vi "USB6363_Output_demo.vi"() -> ()   [LabVIEW 2013]
doc: "This example demonstrates how to continuously re-generate analog output data from a buffer in your computer's memory.\n\nRefer to your device documentation for pinouts and hardware capabilities."
uses:
  <vilib>/Utility/error.llb/DialogType.ctl
  <vilib>/DAQmx/create/channels.llb/DAQmx Create Channel (AO-Voltage-Basic).vi
  <vilib>/DAQmx/configure/timing.llb/DAQmx Timing (Sample Clock).vi
  <vilib>/DAQmx/write.llb/DAQmx Write (Analog 1D Wfm NChan NSamp).vi
  <vilib>/DAQmx/configure/trigger.llb/DAQmx Start Trigger (Digital Edge).vi
  <vilib>/DAQmx/configure/trigger.llb/DAQmx Start Trigger (Analog Edge).vi
  <resource>/objmgr/daqmx.rc
panel:
  in  "Waveform settings":T1={"Tx"=0.3, "Vx_max"=1.0, "Vy_max"=1.0, "Row_N"=20, "ratio of decline"=0.3}
  in  "Trigger Type":T2(tab)
  in  "Edge":i32(ring)=10280 items=["Rising"=10280, "Falling"=10171]
  in  "Digital Trigger Source":tag
  in  "Level (V)":dbl format="%0.2f"
  in  "Hysteresis (V)":dbl
  in  "Slope":i32(ring)=10280 items=["Rising"=10280, "Falling"=10171]
  in  "Analog Trigger Source":string="APFI0"
  in  "Pause When":i32(ring)=10192 items=["High"=10192, "Low"=10214]
  in  "Pause Trigger Source":tag
  in  "Stop":bool
  out "Waveform Graph":waveform(dbl)[](graph)
  in  "Sample Rate":dbl=1000.0
  in  "Sample Clock Source":tag="OnboardClock"
  in  "Max Voltage":dbl=5.0
  in  "Min Voltage":dbl=-5.0
  in  "Physical Channel(s)":tag="Dev1/ao2:3"
  out "Actual Sample Rate":dbl=1000.0 format="%0.2f"
  # "Channel Settings"
  # "Output"
  # "Timing and Buffer Settings"
  # "Trigger Settings"
  # "Waveform Settings"
  # "The number of elements in the waveform array must equal the number of channels in the task."
  # "To configure and use a start trigger you must have the necessary tab selected above.  Not all hardware supports triggering--refer to your device documentation for more info."
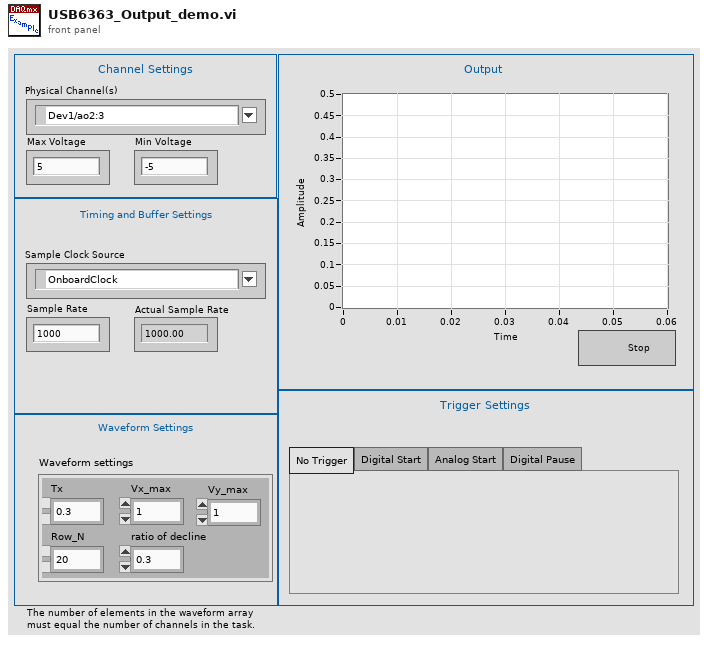
[diagram p1: front panel]
types:
  T1 = cluster{"Tx":dbl, "Vx_max":dbl, "Vy_max":dbl, "Row_N":i32, "ratio of decline":dbl}
  T2 = enum32{"No Trigger", "Digital Start", "Analog Start", "Digital Pause"}
  T3 = typedef "DialogType.ctl" = u16
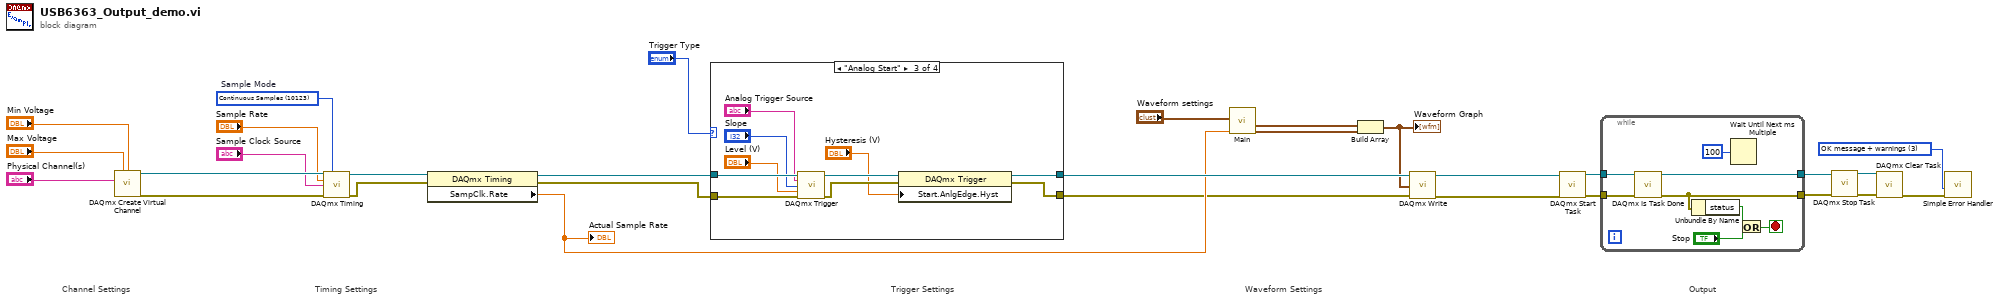
[diagram p0: block diagram]
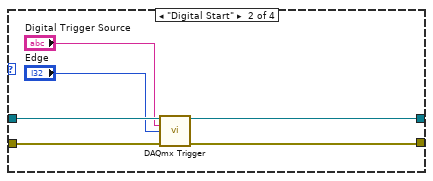
[diagram p3: hidden frame]
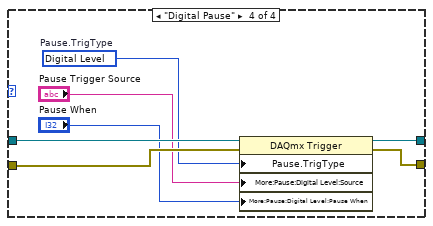
[diagram p4: hidden frame]
diagram:
  w7 = T3 3 items=["no dialog", "OK message", "continue or stop message", "OK message + warnings", "continue/stop + warnings"] ("type of dialog (OK msg:1)")
  w28 = 10123 items=["Finite Samples"=10178, "Continuous Samples"=10123, "Hardware Timed Single Point"=12522]  # Sample Mode
  # "Output"
  # "Trigger Settings"
  # "Waveform Settings"
  # "Timing Settings"
  # "Channel Settings"
  n1 = call-poly <vilib>:"DAQmx Create Virtual Channel.vi"("maximum value"="Max Voltage", "minimum value"="Min Voltage", "physical channels"="Physical Channel(s)") -> ("task out"=w26:refnum<k21>, "error out"=w27:errorcluster)  [unwired: 11 in]
  n2 = call-poly <vilib>:"DAQmx Timing.vi"("task/channels in"=w26, "sample mode"=w28, "rate"="Sample Rate", "source"="Sample Clock Source", "error in"=w27) -> ("task out"=w30:refnum<k21>, "error out"=w29:errorcluster)  [unwired: 9 in]
  n3 = property class="DAQmx Timing"(reference=w30, error in=w29) -> (reference out=w16:refnum<k21>, error out=w15:errorcluster, "SampClk.Rate"=w5:dbl)
  "Actual Sample Rate" <- w5
  n4 = case shown="\"Analog Start\"" "Trigger Type" {
    tunnel: w16 -> [w32 w38 w48 w55]
    tunnel: w15 -> [w31 w37 w47 w52]
    tunnel: [w32 w36 w45 w54] -> w14
    tunnel: [w31 w35 w44 w53] -> w1
    frame "No Trigger", Default {
    }
    frame "Digital Start" {
      n5 = call-poly <vilib>:"DAQmx Trigger.vi"("task/channels in"=w38, "source"="Digital Trigger Source", "edge"="Edge", "error in"=w37) -> ("task out"=w36:refnum<k21>, "error out"=w35:errorcluster)  [unwired: 10 in]
    }
    frame "Analog Start" {
      n6 = call-poly <vilib>:"DAQmx Trigger.vi"("task/channels in"=w48, "source"="Analog Trigger Source", "slope"="Slope", "level"="Level (V)", "error in"=w47) -> ("task out"=w43:refnum<k21>, "error out"=w42:errorcluster)  [unwired: 9 in]
      n7 = property class="DAQmx Trigger"(reference=w43, error in=w42, "Start.AnlgEdge.Hyst"="Hysteresis (V)") -> (reference out=w45:refnum<k21>, error out=w44:errorcluster)
    }
    frame "Digital Pause" {
      w51 = 10152 items=["Analog Level"=10101, "Analog Window"=10103, "Digital Level"=10152, "Digital Pattern"=10398, "None"=10230]  # Pause.TrigType
      n8 = property class="DAQmx Trigger"(reference=w55, error in=w52, "Pause.TrigType"=w51, "More:Pause:Digital Level:Source"="Pause Trigger Source", "More:Pause:Digital Level:Pause When"="Pause When") -> (reference out=w54:refnum<k21>, error out=w53:errorcluster)
    }
  }
  n9 = call "Main.vi"("Fs (Hz)"=w5, "Waveform settings"="Waveform settings") -> ("Y"=w3:waveform(dbl), "X"=w4:waveform(dbl))  [unwired: 7 in, 1 out]
  n10 = Build Array(w4, w3) -> (w2:waveform(dbl)[])
  "Waveform Graph" <- w2
  n11 = call-poly <vilib>:"DAQmx Write.vi"("task/channels in"=w14, "data"=w2, "error in"=w1) -> ("task out"=w13:refnum<k21>, "error out"=w12:errorcluster)  [unwired: 10 in, 1 out]
  n12 = call <vilib>:"DAQmx Start Task.vi"("task/channels in"=w13, "error in"=w12) -> ("task out"=w25:refnum<k21>, "error out"=w24:errorcluster)  [unwired: 12 in]
  n13 = while {
    tunnel: w25 -> [w63]
    tunnel: w24 -> [w62]
    tunnel: [w59] -> w8
    tunnel: [w60] -> w9
    stop <- w61 stop-if-true
    n14 = call <vilib>:"DAQmx Is Task Done.vi"("task/channels in"=w63, "error in"=w62) -> ("task out"=w60:refnum<k21>, "error out"=w59:errorcluster)  [unwired: 11 in, 1 out]
    n15 = Unbundle By Name(w59) -> ("status"=w58:bool)
    n16 = Wait Until Next ms Multiple(millisecond multiple=u32 100) -> ()  [unwired: 1 out]
    n17 = Or(x=w58, y="Stop") -> (x .or. y?=w61:bool)
  }
  n18 = call <vilib>:"DAQmx Stop Task.vi"("task/channels in"=w9, "error in"=w8) -> ("task out"=w11:refnum<k21>, "error out"=w10:errorcluster)  [unwired: 12 in]
  n19 = call <vilib>:"DAQmx Clear Task.vi"("task in"=w11, "error in"=w10) -> ("error out"=w23:errorcluster)  [unwired: 13 in]
  n20 = call <vilib>:"Simple Error Handler.vi"("type of dialog (OK msg:1)"=w7, "error in (no error)"=w23) -> ()  [unwired: 3 in, 5 out]
